vi "TestExecuteWriteWhenVisibleSubscription_UpdateOK.vi"(8 "error in (no error)":errorcluster, 11 "TestCase in":refnum<class "TestSubscriptionPolicy.lvclass">) -> (0 "error out":errorcluster, 3 "TestCase out":refnum<class "TestSubscriptionPolicy.lvclass">)   [LabVIEW 2017, in "TestSubscriptionPolicy.lvclass"]
uses:
  TestSubscriptionPolicy.lvclass
  Source/Framework/IMediator/ISubscriptionPolicy/ISubscriptionPolicy.lvclass/ISubscriptionPolicy.ctl
  Source/Framework/SubscriptionPolicy/WriteWhenVisibleSubscription/WriteWhenVisibleSubscription.lvclass
  C:/Git/mva-framework/Source/Framework/IMediator/ISubscriptionPolicy/ISubscriptionPolicy.lvclass
  Source/Framework/Transport/TerminalBinding/TerminalBinding.lvclass
  C:/Git/mva-framework/Source/Framework/IMediator/ITransport/ITransport.lvclass
  Source/Framework/IMediator/ISubscriptionPolicy/ISubscriptionPolicy.lvclass
panel:
  in  "Numeric":dbl
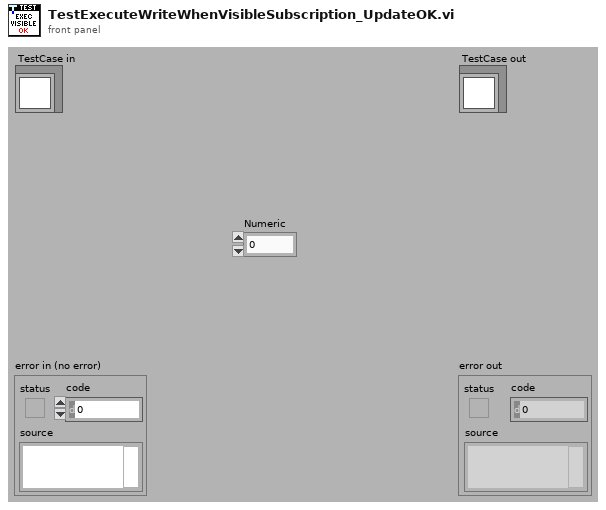
[diagram p1: front panel]
types:
  T1 = typedef "IMediator.lvlib/ISubscriptionPolicy.lvclass/ISubscriptionPolicy Reference.ctl" = refnum<data-value>
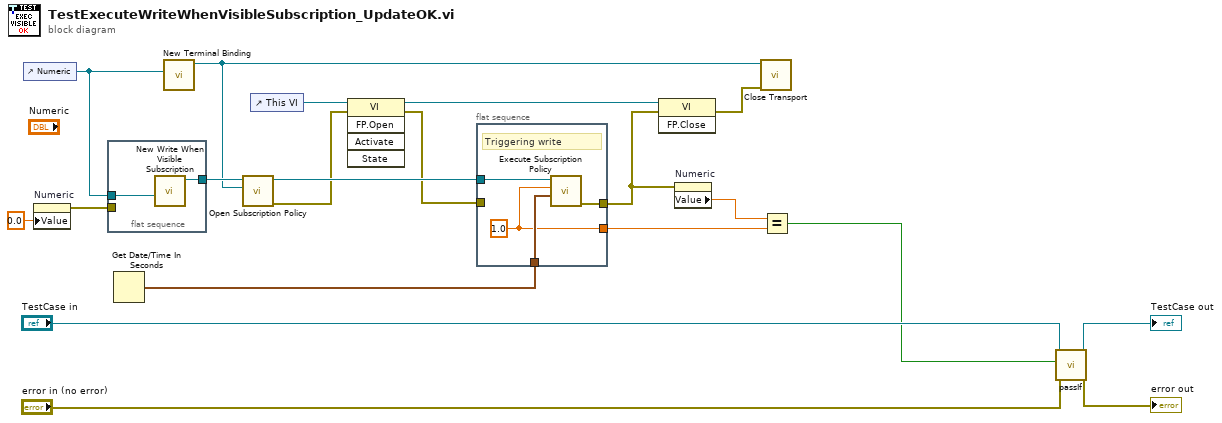
[diagram p0: block diagram]
diagram:
  n1 = control-ref of="Numeric"() -> (w2:refnum<vi>)
  n2 = property on="Numeric" class="DigNum (strict)"("Value"=0.0 ("Numeric")) -> (error out=w5:errorcluster)  [unwired: 2 in, 1 out]
  n3 = flat-sequence {
    tunnel: [w22] -> w16
    tunnel: w5 -> [_]
    tunnel: w2 -> [w21]
    frame #0 {
      n4 = call "New Write When Visible Subscription.vi"("Ctl Refnum"=w21) -> ("WriteWhenVisibleSubscription Out"=w22:refnum<class "WriteWhenVisibleSubscription.lvclass">)  [unwired: 10 in]
    }
  }
  n5 = Get Date/Time In Seconds() -> (seconds since 1Jan1904=w12:timestamp)
  n6 = call "New Terminal Binding.vi"("Ctl Refnum"=w2) -> ("TerminalBinding"=w13:refnum<class "TerminalBinding.lvclass">)  [unwired: 9 in, 1 out]
  n7 = call "Open Subscription Policy.vi"("Transport"=w13, "SubscriptionPolicy"=w16) -> ("error out"=w10:errorcluster, "Subscription Policy"=w15:T1)  [unwired: 8 in]
  n8 = control-ref of="This VI"() -> (w11:refnum<vi>)
  n9 = invoke class="VI" method="FP.Open"(reference=w11, error in=w10) -> (reference out=w8:refnum<vi>, error out=w9:errorcluster)  [unwired: 3 in, 3 out]
  n10 = flat-sequence {
    tunnel: w15 -> [w26]
    tunnel: w12 -> [w25]
    tunnel: [w24] -> w4
    tunnel: [w23] -> w14
    tunnel: w9 -> [_]
    frame #0 {
      w23 = 1.0
      # "Triggering write"
      n11 = call "Execute Subscription Policy.vi"("Publish Time"=w25, "New Topic Value"=w23, "Subscription Policy"=w26) -> ("error out (Unsubscribe?)"=w24:errorcluster)  [unwired: 7 in, 1 out]
    }
  }
  n12 = invoke class="VI" method="FP.Close"(reference=w8, error in=w4) -> (error out=w7:errorcluster)  [unwired: 1 in, 2 out]
  n13 = property on="Numeric" class="DigNum (strict)"(error in=w4) -> ("Value"=w3:dbl)  [unwired: 1 in, 2 out]
  n14 = call-dynamic "Close Transport.vi"("error in (no error)"=w7, "ITransport in"=w13) -> ()  [unwired: 9 in, 1 out]
  n15 = Equal?(x=w3, y=w14) -> (x = y?=w1:bool)
  n16 = call-dynamic "passIf.vi"("error in (no error)"="error in (no error)", "pass"=w1, "TestCase in"="TestCase in") -> ("error out"=→"error out":errorcluster, "TestCase out"=→"TestCase out":refnum<class "TestSubscriptionPolicy.lvclass">)  [unwired: 7 in]
